vi "Nanonis_SR830_ExternalDevice_Single.vi"() -> ()   [LabVIEW 2021]
uses:
  <instrlib>/Stanford Research 830/Public/Data/Read (All Parameters).vi
  <instrlib>/Stanford Research 830/Stanford Research 830.lvlib
panel:
  in  "Polling Time (ms)":u32
  in  "program_stop":bool
  in  "System Reset All?":bool
  out "Reference Freq":dbl
  out "Theta-Value":dbl
  out "R-Value":dbl
  out "X-Value":dbl
  in  "SR830 #1\nSensitivity":i16(ring)=17 items=["Auto Gain"=-1, "2 nV/fA"=0, "5 nV/fA"=1, "10 nV/fA"=2, "20 nV/fA"=3, "50 nV/fA"=4, "100 nV/fA"=5, "200 nV/fA"=6, "500 nV/fA"=7, "1 uV/pA"=8, "2 uV/pA"=9, "5 uV/pA"=10, "10 uV/pA"=11, "20 uV/pA"=12, "50 uV/pA"=13, "100 uV/pA"=14, "200 uV/pA"=15, "500 uV/pA"=16, "1 mV/nA"=17, "2 mV/nA"=18, "5 mV/nA"=19, "10 mV/nA"=20, "20 mV/nA"=21, "50 mV/nA"=22, "100 mV/nA"=23, "200 mV/nA"=24, "500 mV/mA"=25, "1 V/uA"=26]
  in  "SR830 #1 \nDynamic Reserve":i16(ring)=1 items=["Auto Reserve"=-1, "High Reserve"=0, "Normal"=1, "Low Noise"=2]
  in  "SR830 #1\nSync Filter":bool
  in  "SR830 #1 Low\nPass Filter Slope":u16(ring)=3 items=["6 dB/oct", "12 dB/oct", "18 db/oct", "24 dB/oct"]
  in  "SR830 #1 \nTime Constant":u16(ring)=8 items=["10 us", "30 us", "100 us", "300 us", "1 ms", "3 ms", "10 ms", "30 ms", "100 ms", "300 ms", "1 s", "3 s", "10 s", "30 s", "100 s", "300 s", "1 ks", "3 ks", "10 ks", "30 ks"]
  in  "SR830 #1 \nAuto Phase":bool
  in  "SR830 #1 Manual \nPhase":dbl
  in  "SR830 #1 Reference Source":u16(ring)=1 items=["External", "Internal"]
  in  "SR830 #1 Sine \nOutput Amplitude":dbl=1.0
  in  "SR830 #1 Detection Harm. Num.":dbl=1.0
  in  "SR830 #1 Internal \nReference Frequency":dbl=17.0
  in  "SR830 #1 Trigger Source":u16(ring) items=["Internal", "External"]
  in  "SR830 #1 Input\nNotch Filter":u16(ring) items=["None", "Line Notch", "2x Line Notch", "Both Notch Filters"]
  in  "SR830 #1 Input \nShield Grounding":u16(ring) items=["Float", "Ground"]
  in  "SR830 #1\nInput Coupling":u16(ring) items=["AC", "DC"]
  in  "SR830 #1 Input Connection":u16(ring)=1 items=["Single-Ended Voltage", "Differential Voltage", "1 MOhm Current Gain", "100 MOhm Current Gain"]
  in  "SR830 #1":refnum<visa-resource-name>="GPIB0::10::INSTR"
  in  "System #1 Enabled/Disabled":bool
  # "SR830"
  # "Input Signal"
  # "Readout (Recorded)"
  # "Source / Reference"
  # "Input Filters & Sens"
  # "Initialisation:\n--> Reset \n--> Instruments?"
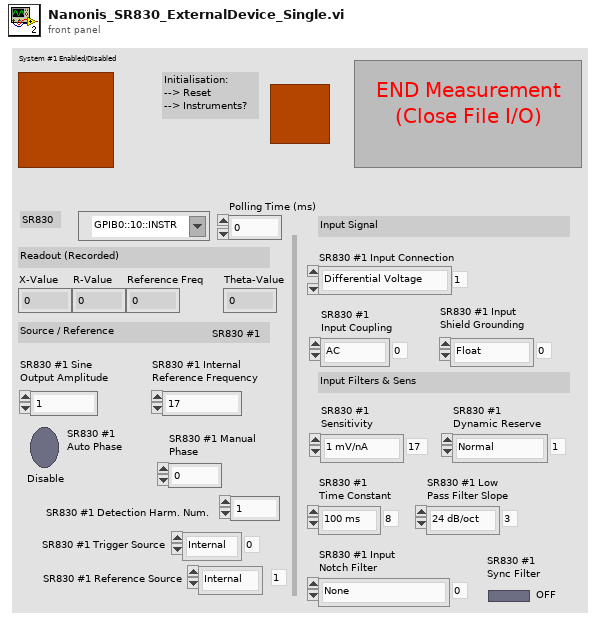
[diagram p1: front panel]
types:
  T1 = cluster{"VISA resource name out":refnum<visa-resource-name>, "error out":errorcluster}
  T2 = cluster{cluster{"VISA resource name out":refnum<visa-resource-name>, "error out":errorcluster}}
  T3 = cluster{"X-Value":dbl, "Y-Value":dbl, "R-Value":dbl, "Theta-Value":dbl, "Aux In 1 Value":dbl, "Aux In 2 Value":dbl, "Aux In 3 Value":dbl, "Aux In 4 Value":dbl, "Reference Frequency":dbl, "Channel 1 Display":dbl, "Channel 2 Display":dbl}
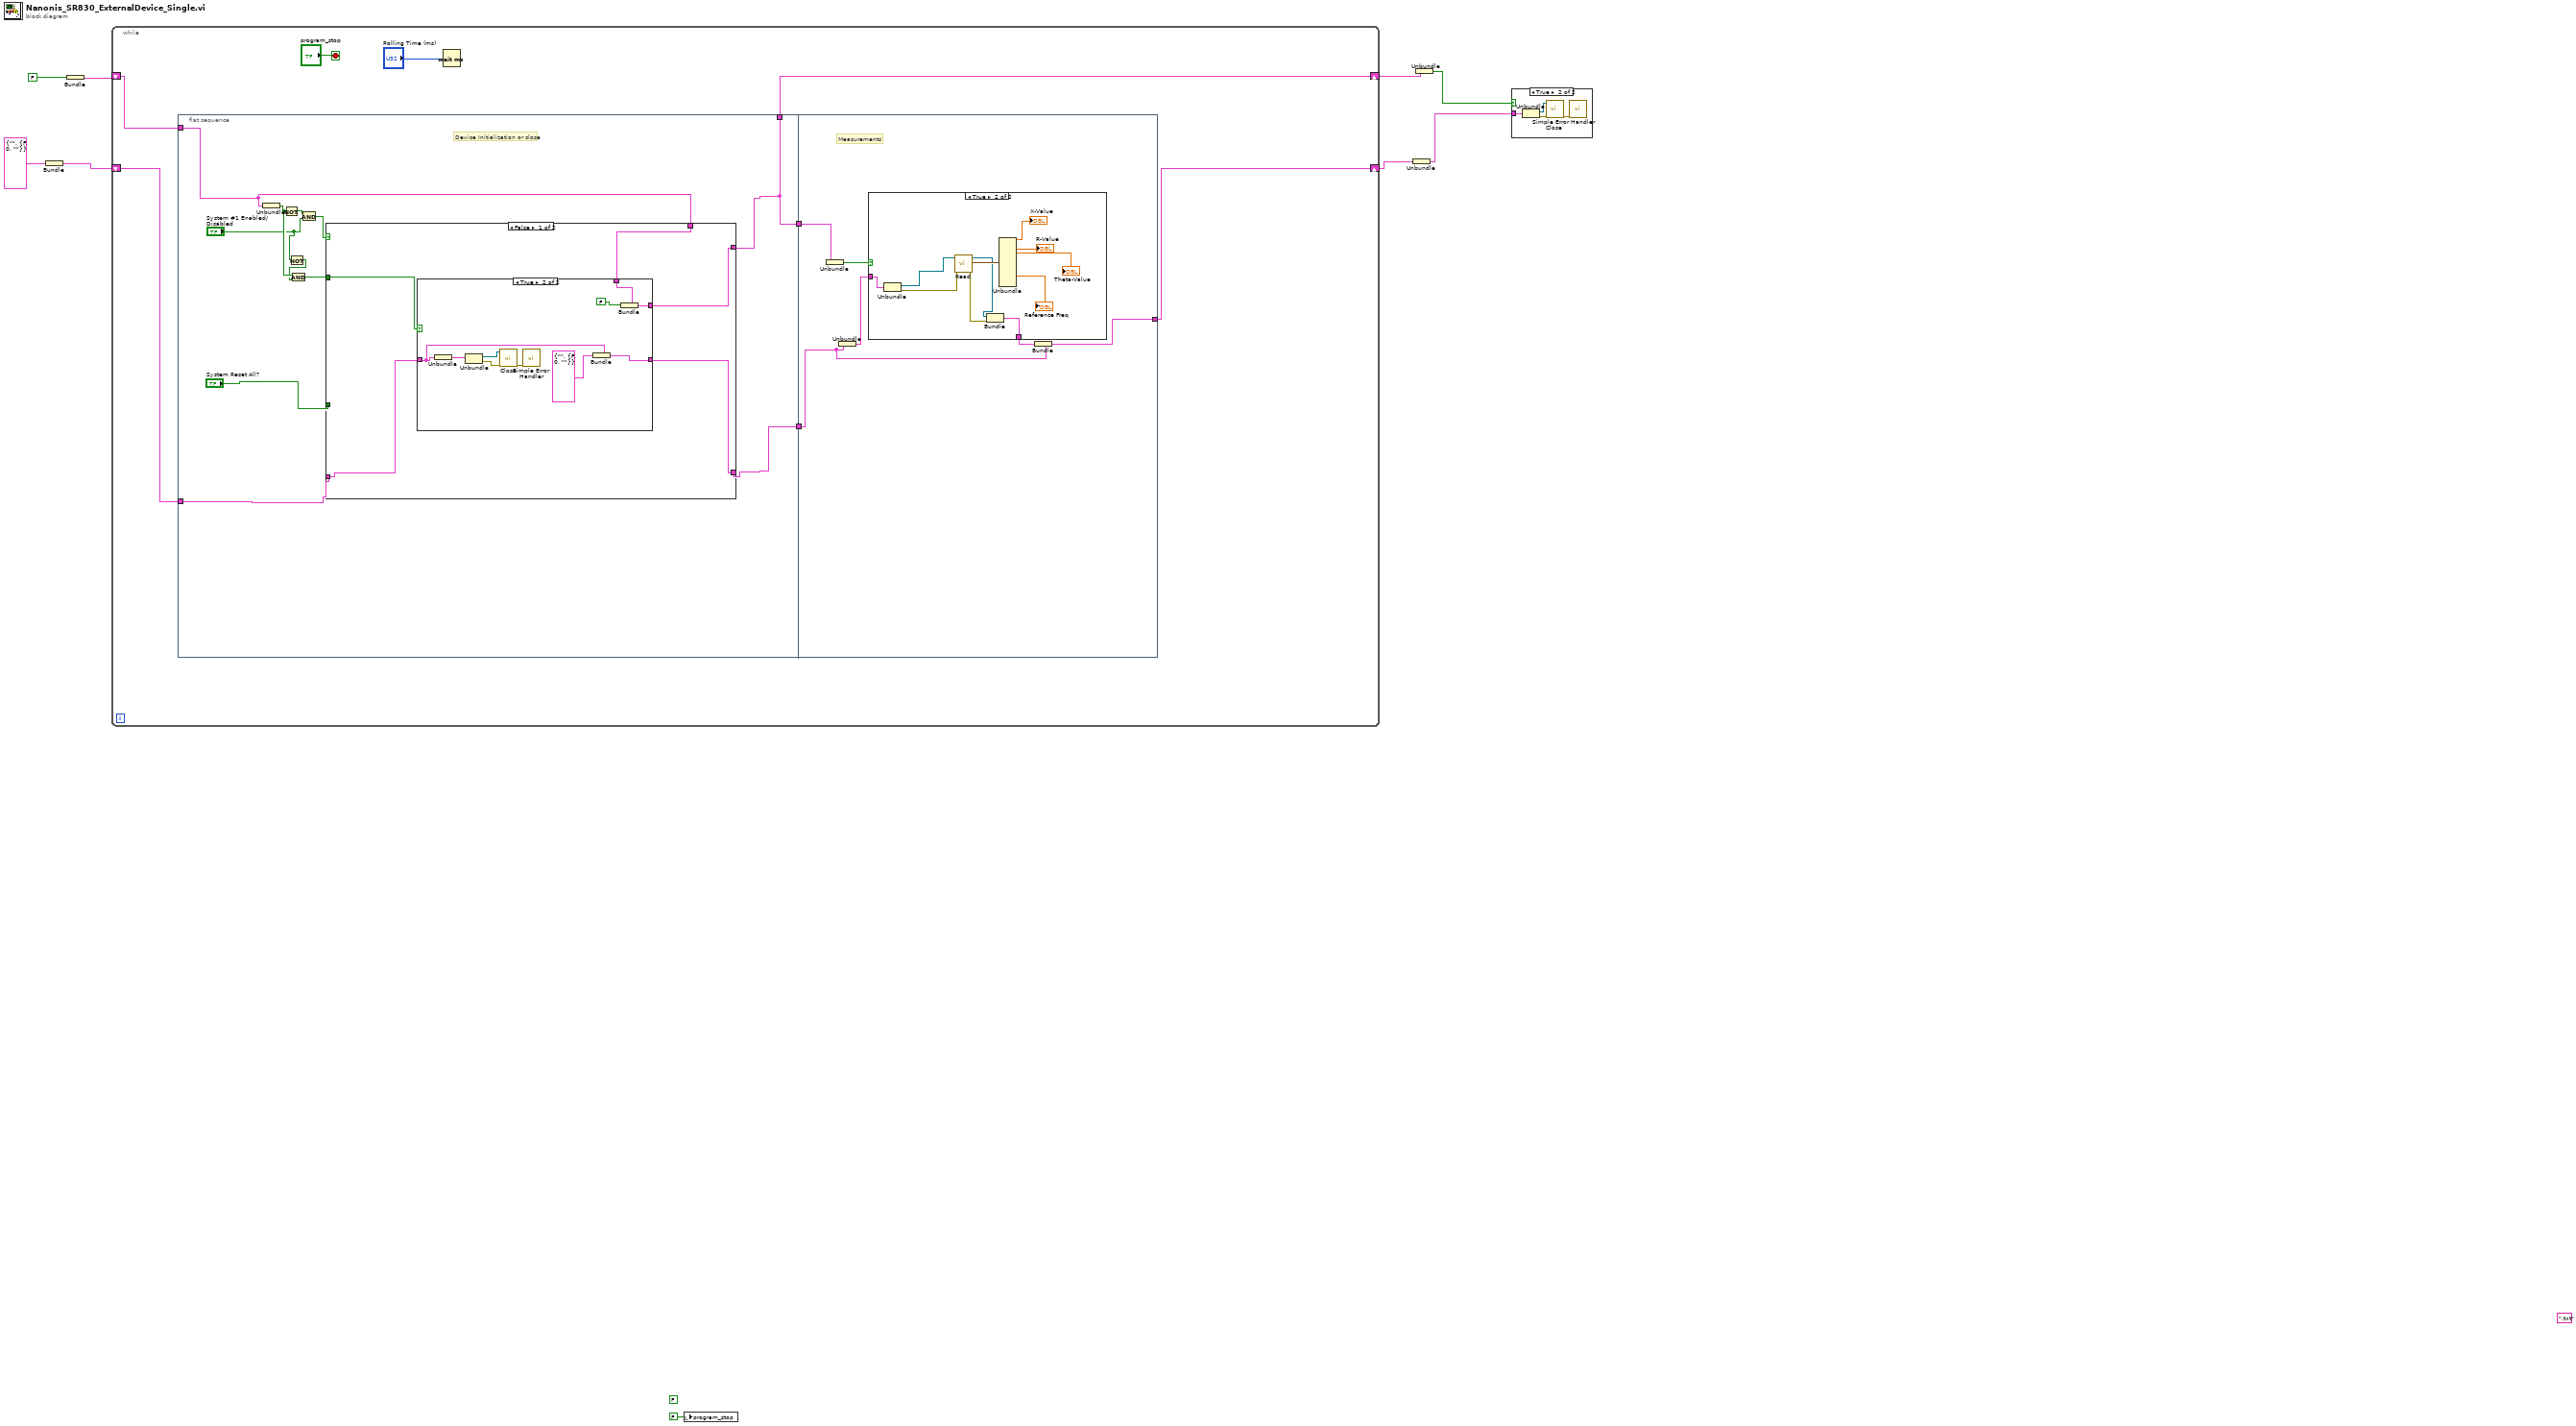
[diagram p0: block diagram]
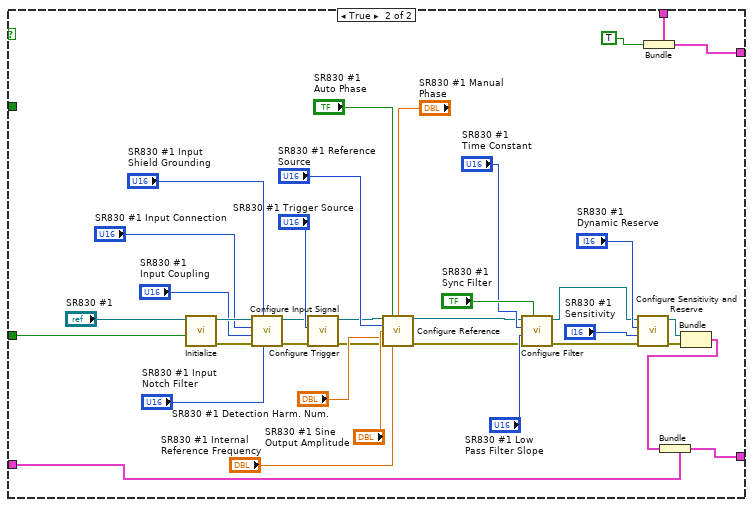
[diagram p4: hidden frame]
diagram:
  (unwired) ".txt"
  (unwired) FALSE ("Measuring")
  n1 = Bundle(T1 {"VISA resource name out"="", "error out"={"status"=FALSE, "code"=0, "source"=""}}) -> (w5:T2)  [unwired: 1 in]
  n2 = Bundle(FALSE) -> (w7:cluster{bool})  [unwired: 1 in]
  n3 = while {
    shift-right: [w12] -> w4
    shift-left: w7 -> [w16]
    shift-right: [w11] -> w3
    shift-left: w5 -> [w15]
    stop <- "program_stop" stop-if-true
    n4 = flat-sequence {
      tunnel: w16 -> [w27]
      tunnel: w15 -> [w26]
      tunnel: [w23] -> w14
      tunnel: [w22] -> w13
      tunnel: [w22] -> w12
      tunnel: w14 -> [w82]
      tunnel: w13 -> [w87]
      tunnel: [w83] -> w11
      frame #0 {
        # "Device Initialization or close"
        n5 = Unbundle(w27) -> (w21:bool)
        n6 = Not(x=w21) -> (.not. x?=w25:bool)
        n7 = Not(x="System #1 Enabled/Disabled") -> (.not. x?=w18:bool)
        n8 = And(x=w21, y=w18) -> (x .and. y?=w20:bool)
        n9 = And(x=w25, y="System #1 Enabled/Disabled") -> (x .and. y?=w24:bool)
        n10 = case shown="False" w24 {
          tunnel: "System Reset All?" -> [_ w52]
          tunnel: w27 -> [w30 w51]
          tunnel: [w29 w50] -> w22
          tunnel: w26 -> [w33 w48]
          tunnel: [w32 w46] -> w23
          tunnel: w20 -> [w31 _]
          frame False {
            n11 = case shown="True" w31 {
              tunnel: w33 -> [w35 w42]
              tunnel: [w35 w40] -> w32
              tunnel: w30 -> [w34 w37]
              tunnel: [w34 w36] -> w29
              frame False {
              }
              frame True {
                n12 = Unbundle(w42) -> (w39:T1)
                n13 = Unbundle(w39) -> ("VISA resource name out"=w44:refnum<visa-resource-name>, "error out"=w43:errorcluster)
                n14 = call <instrlib>:"Close.vi"("error in (no error)"=w43, "VISA resource name"=w44) -> ("error out"=w45:errorcluster)  [unwired: 9 in]
                n15 = call <vilib>:"Simple Error Handler.vi"("error in (no error)"=w45) -> ()  [unwired: 4 in, 5 out]
                n16 = Bundle(cluster=w42, T1 {"VISA resource name out"="", "error out"={"status"=FALSE, "code"=0, "source"=""}}) -> (w40:T2)
                n17 = Bundle(cluster=w37, FALSE) -> (w36:cluster{bool})
              }
            }
          }
          frame True {
            n18 = call <instrlib>:"Initialize.vi"("Reset (True)"=w52, "VISA resource name"="SR830 #1") -> ("error out"=w57:errorcluster, "VISA resource name out"=w56:refnum<visa-resource-name>)  [unwired: 8 in]
            n19 = call <instrlib>:"Configure Input Signal.vi"("Input Notch Filter (0: None)"="SR830 #1 Input\nNotch Filter", "Input Shield Grounding (0: Float)"="SR830 #1 Input \nShield Grounding", "error in (no error)"=w57, "Input Coupling (0: AC)"="SR830 #1\nInput Coupling", "Input Connection (0: Single-Ended Voltage)"="SR830 #1 Input Connection", "VISA resource name"=w56) -> ("error out"=w59:errorcluster, "VISA resource name out"=w58:refnum<visa-resource-name>)  [unwired: 4 in]
            n20 = call <instrlib>:"Configure Trigger.vi"("error in (no error)"=w59, "Trigger Source (0: Internal)"="SR830 #1 Trigger Source", "VISA resource name"=w58) -> ("error out"=w61:errorcluster, "VISA resource name out"=w60:refnum<visa-resource-name>)  [unwired: 7 in]
            n21 = call <instrlib>:"Configure Reference.vi"("VISA resource name"=w60, "Auto Phase (T: Enabled)"="SR830 #1 \nAuto Phase", "Manual Phase (0 Degree)"="SR830 #1 Manual \nPhase", "Reference Source (1: Internal)"="SR830 #1 Reference Source", "Sine Output Amplitude (1 V)"="SR830 #1 Sine \nOutput Amplitude", "Detection Harmonic Number (1)"="SR830 #1 Detection Harm. Num.", "error in (no error)"=w61, "Internal Reference Frequency (1000 Hz)"="SR830 #1 Internal \nReference Frequency") -> ("VISA resource name out"=w63:refnum<visa-resource-name>, "error out"=w62:errorcluster)  [unwired: 6 in]
            n22 = call <instrlib>:"Configure Filter.vi"("Enable Sync Filter (F: Disable)"="SR830 #1\nSync Filter", "error in (no error)"=w62, "Low Pass Filter Slope (1: 12dB/oct)"="SR830 #1 Low\nPass Filter Slope", "Time Constant (8: 100ms)"="SR830 #1 \nTime Constant", "VISA resource name"=w63) -> ("error out"=w77:errorcluster, "VISA resource name out"=w76:refnum<visa-resource-name>)  [unwired: 5 in]
            n23 = call <instrlib>:"Configure Sensitivity and Reserve.vi"("error in (no error)"=w77, "Sensitivity (-1: Auto gain)"="SR830 #1\nSensitivity", "Dynamic Reserve (-1: Auto Reserve)"="SR830 #1 \nDynamic Reserve", "VISA resource name"=w76) -> ("error out"=w81:errorcluster, "VISA resource name out"=w80:refnum<visa-resource-name>)  [unwired: 6 in]
            n24 = Bundle(cluster=w51, TRUE) -> (w50:cluster{bool})
            n25 = Bundle("VISA resource name out"=w80, "error out"=w81) -> (w47:T1)  [unwired: 1 in]
            n26 = Bundle(cluster=w48, w47) -> (w46:T2)
          }
        }
      }
      frame #1 {
        # "Measurements"
        n27 = Unbundle(w87) -> (w86:bool)
        n28 = Unbundle(w82) -> (w84:T1)
        n29 = case shown="True" w86 {
          tunnel: [w88 w94] -> w85
          tunnel: w84 -> [w88 w93]
          frame False {
          }
          frame True {
            n30 = Unbundle(w93) -> ("VISA resource name out"=w99:refnum<visa-resource-name>, "error out"=w98:errorcluster)
            n31 = call-poly <instrlib>:"Read.vi"("error in (no error)"=w98, "VISA resource name"=w99) -> ("error out"=w96:errorcluster, "Parameter Values"=w97:T3, "VISA resource name out"=w95:refnum<visa-resource-name>)  [unwired: 7 in]
            n32 = Bundle("VISA resource name out"=w95, "error out"=w96) -> (w94:T1)  [unwired: 1 in]
            n33 = Unbundle(w97) -> ("X-Value"=→"X-Value":dbl, "R-Value"=→"R-Value":dbl, "Theta-Value"=→"Theta-Value":dbl, "Reference Frequency"=→"Reference Freq":dbl)  [unwired: 7 out]
          }
        }
        n34 = Bundle(cluster=w82, w85) -> (w83:T2)
      }
    }
    n35 = Wait (ms)(milliseconds to wait="Polling Time (ms)") -> ()  [unwired: 1 out]
  }
  n36 = local write "program_stop"(FALSE ("program_stop")) -> ()
  n37 = Unbundle(w3) -> (w1:T1)
  n38 = Unbundle(w4) -> (w2:bool)
  n39 = case shown="True" w2 {
    tunnel: w1 -> [_ w100]
    frame False {
    }
    frame True {
      n40 = Unbundle(w100) -> ("VISA resource name out"=w102:refnum<visa-resource-name>, "error out"=w101:errorcluster)
      n41 = call <instrlib>:"Close.vi"("error in (no error)"=w101, "VISA resource name"=w102) -> ("error out"=w103:errorcluster)  [unwired: 9 in]
      n42 = call <vilib>:"Simple Error Handler.vi"("error in (no error)"=w103) -> ()  [unwired: 4 in, 5 out]
    }
  }
